vi "ScoreControl.vi"(0 "Get/Set Mode Selector":u16(ring) items=["Get All", "Set", "Reset All", "Force Set", "Force Set All"], 5 "Full Score Entry":T3={"Elements"=[{"Name"="CO2 Balls Touching/Within Reservoir Model", "Value"="-1"}, {"Name"="Money Ball Touching/Within Reservoir Model", "Value"="-1"}, {"Name"="3+ Red/White Citizens in Pink Grid Area", "Value"="-1"}, {"Name"="# Upright Levee Blocks touching ONLY GREEN shores", "Value"="-1"}, {"Name"="# Upright Levee Blocks Touching any RED shore", "Value"="-1"}, {"Name"="Levee Test was Performed", "Value"="-1"}, {"Name"="Levee Test Wheel Blocked by NonLevee", "Value"="-1"}, {"Name"="Flood Barrier in Up Position", "Value"="-1"}, {"Name"="Both Yellow Arrows Aligned", "Value"="-1"}, {"Name"="Team Robot Touching Only Yellow Grid Area", "Value"="-1"}, {"Name"="Both Insulation Touching Green Grid Area", "Value"="-1"}, {"Name"="Bicycle Touching Green Grid Area", "Value"="-1"}, {"Name"="Computer Touching Green Grid Area", "Value"="-1"}, {"Name"="House in Up Position", "Value"="-1"}, {"Name"="House Window Showing Black", "Value"="-1"}, {"Name"="House Window All The Way Open", "Value"="-1"}, {"Name"="3+ Black/White Scientists Touching Research Area", "Value"="-1"}, {"Name"="Money Ball Touching/Within Research Area Model", "Value"="-1"}, {"Name"="Polar Bear Touching/Within Research Area Model", "Value"="-1"}, {"Name"="Polar Bear Orientation (Sleeping/Upright)", "Value"="-1"}, {"Name"="Ice Core Pulled From Its Hole", "Value"="-1"}, {"Name"="Ice Buoy Upright and Within/Touching Research Area Model", "Value"="-1"}, {"Name"="Drilling Machine Touching/Within Research Area Model", "Value"="-1"}, {"Name"="Drill Assembly Completely Vertical", "Value"="-1"}, {"Name"="Team Robot Touching/Within Research Area Model", "Value"="-1"}, {"Name"="3+ Blue/Gray Leaders Touching Green Mountain/City Area", "Value"="-1"}, {"Name"="Ice Core in Base Area", "Value"="-1"}, {"Name"="Snowmobile Touching/Within Research Area Model", "Value"="-1"}], "Score"=0.0}, 7 "GUID":u16, 9 "Round Number":u16, 11 "Score Mode Selector":u16(ring) items=["Automatic", "Manual"], 12 "All Scores":T1 {"Score"."Score Mode Selector" items=["Automatic", "Manual"]}) -> (4 "Scores":T1 {"Score"."Score Mode Selector" items=["Automatic", "Manual"]}, 15 "Errors":string)   [LabVIEW 2013]
uses:
  ScoreEntry.ctl
  ScoreList.ctl
  Full Score Entry.ctl
  Score Event Refnum.vi
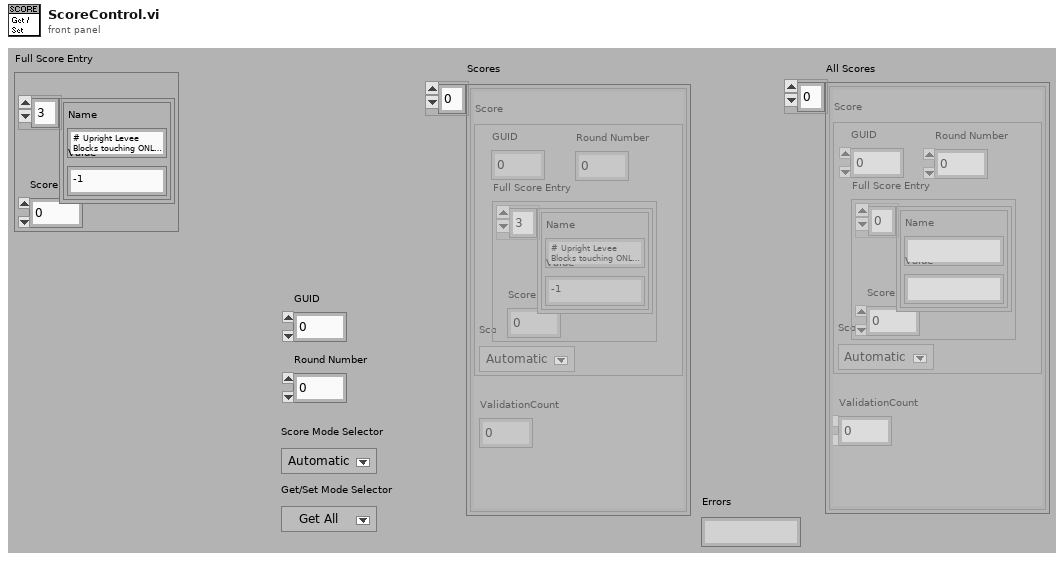
[diagram p1: front panel]
types:
  T1 = typedef "ScoreList.ctl" = cluster{"ValidationCount":u16, "Score":T2}[]
  T2 = typedef "Full Score Entry.ctl" = cluster{"GUID":u16, "Score Mode Selector":u16, "Round Number":u16, "Full Score Entry":T3}
  T3 = typedef "ScoreEntry.ctl" = cluster{"Elements":cluster{"Name":string, "Value":string}[], "Score":dbl}
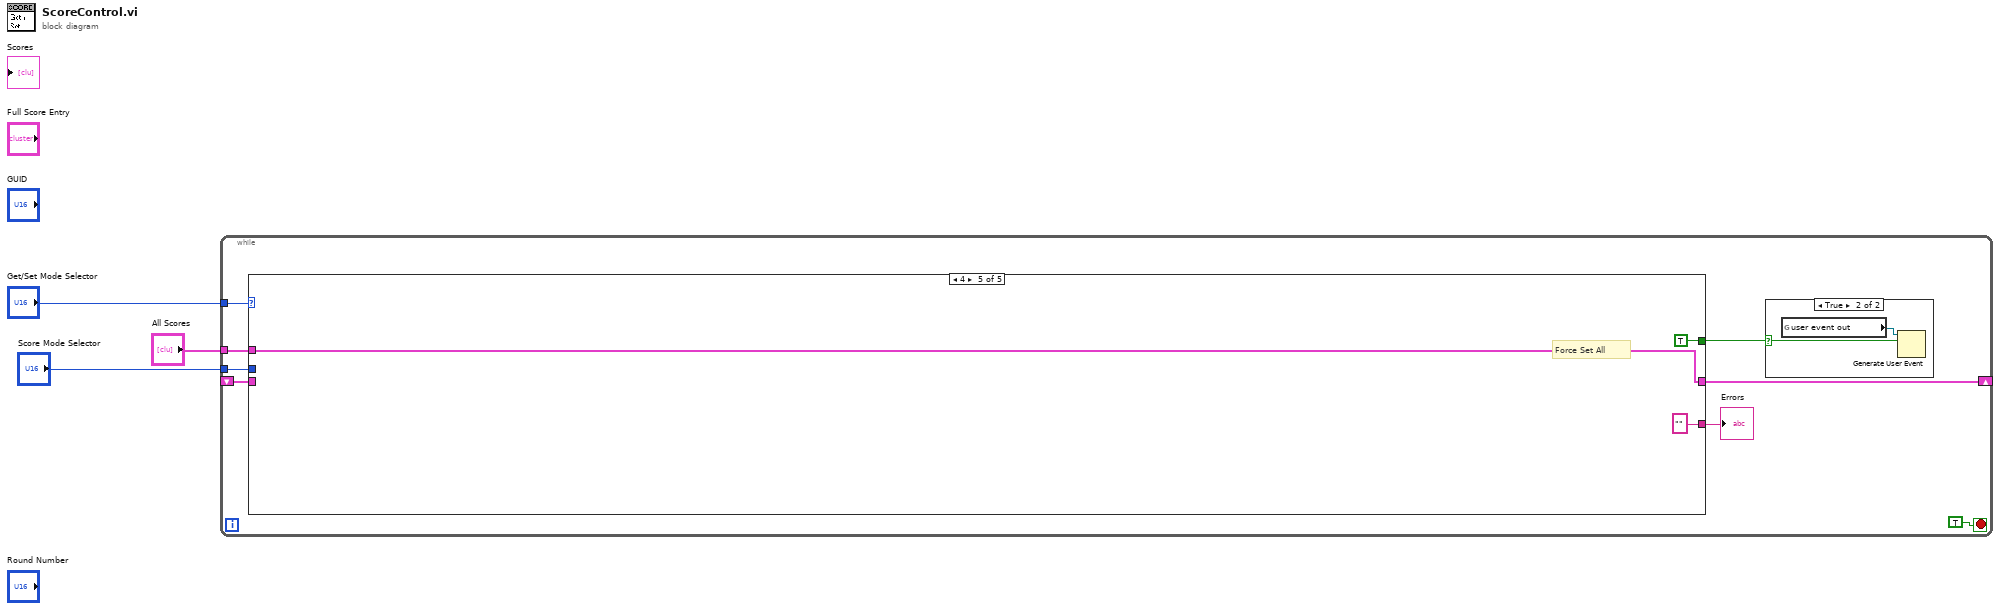
[diagram p0: block diagram]
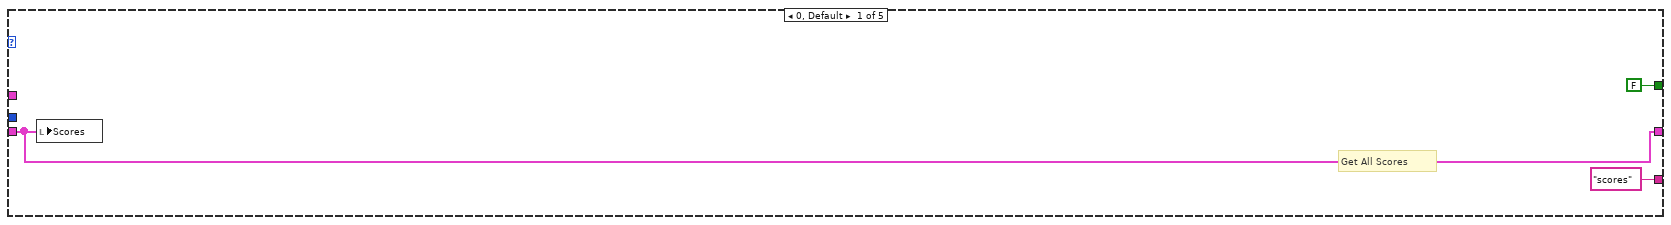
[diagram p3: hidden frame]
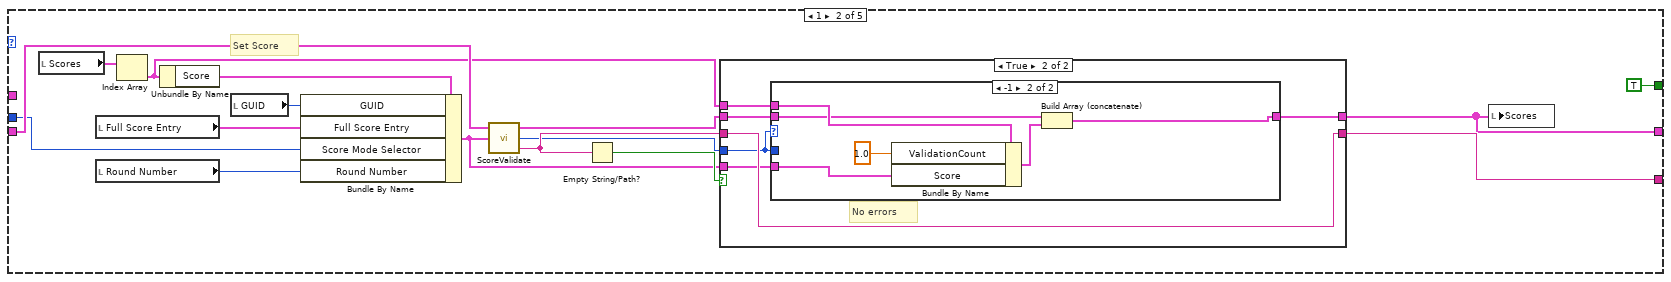
[diagram p4: hidden frame]
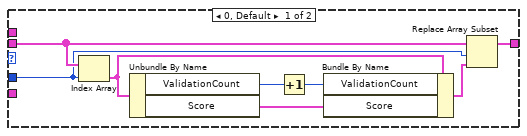
[diagram p6: hidden frame]
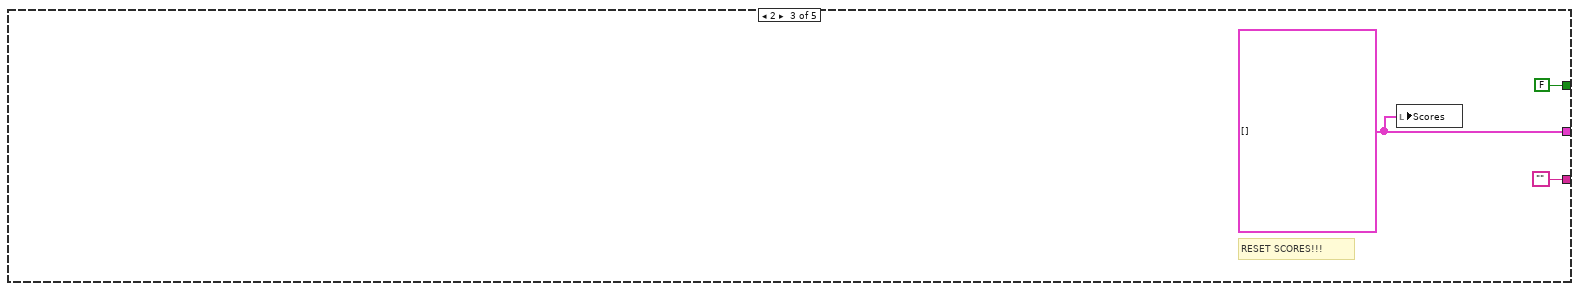
[diagram p7: hidden frame]
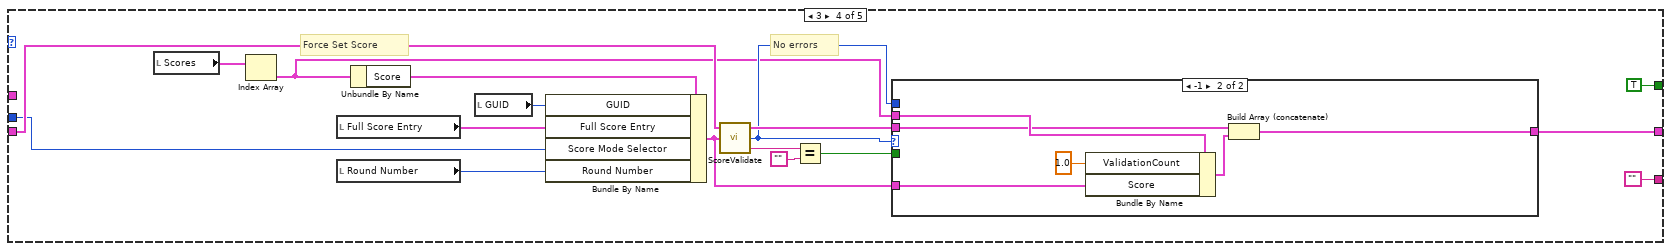
[diagram p8: hidden frame]
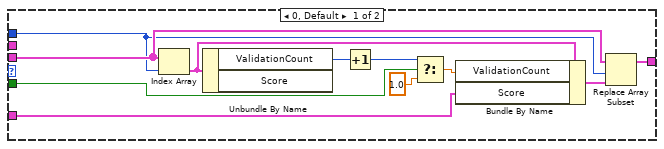
[diagram p9: hidden frame]
diagram:
  n1 = while {
    tunnel: "Get/Set Mode Selector" -> [w11]
    tunnel: "Score Mode Selector" -> [w10]
    shift-right: [w7] -> _
    shift-left: _ -> [w9]
    tunnel: "All Scores" -> [w6]
    stop <- TRUE stop-if-true
    n2 = case shown="4" w11 {
      tunnel: w9 -> [w16 w32 _ w74 _]
      tunnel: [w16 w18 w56 w66 w92] -> w7
      tunnel: ["scores" w31 "" "" "" ("Errors")] -> w5
      tunnel: w10 -> [_ w19 _ w62 _]
      tunnel: w6 -> [_ _ _ _ w92]
      tunnel: [FALSE ("event data") TRUE ("event data") FALSE ("event data") TRUE ("event data") TRUE ("event data")] -> w4
      frame 0, Default {
        # "Get All Scores"
        n3 = local write "Scores"(w16) -> ()
      }
      frame 1 {
        # "Set Score"
        n4 = local read "Scores"() -> (w30:T1)
        n5 = local read "Full Score Entry"() -> (w29:T3)
        n6 = local read "Round Number"() -> (w27:u16)
        n7 = Index Array(array=w30) -> (element=w20:cluster{"ValidationCount":u16, "Score":T2})  [unwired: 1 in]
        n8 = Unbundle By Name(w20) -> ("Score"=w22:T2)
        n9 = local read "GUID"() -> (w28:u16)
        n10 = Bundle By Name(cluster=w22, "GUID"=w28, "Full Score Entry"=w29, "Score Mode Selector"=w19, "Round Number"=w27) -> (w24:T2)
        n11 = call "ScoreValidate.vi"("Score"=w24, "Scores"=w32) -> ("Errors"=w23:string, "Index"=w21:i32, "Scores Out"=w25:T1)  [unwired: 1 in]
        n12 = Empty String/Path?(string/path=w23) -> (empty?=w26:bool)
        n13 = case shown="True" w26 {
          tunnel: w25 -> [w33 w38]
          tunnel: w24 -> [_ w36]
          tunnel: w23 -> [w34 w40]
          tunnel: [w34 w40] -> w31
          tunnel: [w33 w39] -> w18
          tunnel: w21 -> [_ w37]
          tunnel: w20 -> [_ w35]
          frame False {
          }
          frame True {
            # "No errors"
            n14 = case shown="-1" w37 {
              tunnel: [w48 w49] -> w39
              tunnel: w38 -> [w47 w50]
              tunnel: w37 -> [w41 _]
              tunnel: w36 -> [_ w53]
              tunnel: w35 -> [_ w52]
              frame 0, Default {
                n15 = Index Array(array=w47, index=w41) -> (element=w46:cluster{"ValidationCount":u16, "Score":T2})
                n16 = Unbundle By Name(w46) -> ("ValidationCount"=w43:u16, "Score"=w42:T2)
                n17 = Increment(x=w43) -> (x+1=w44:u16)
                n18 = Bundle By Name(cluster=w46, "ValidationCount"=w44, "Score"=w42) -> (w45:cluster{"ValidationCount":u16, "Score":T2})
                n19 = Replace Array Subset(array=w47, new element=w45, index=w41) -> (w48:T1)
              }
              frame -1 {
                n20 = Bundle By Name(cluster=w52, "ValidationCount"=1.0, "Score"=w53) -> (w51:cluster{"ValidationCount":u16, "Score":T2})
                n21 = Build Array (concatenate)(w50, w51) -> (w49:T1)
              }
            }
          }
        }
        n22 = local write "Scores"(w18) -> ()
      }
      frame 2 {
        w56 = T1 [] ("Scores")
        # "RESET SCORES!!!"
        n23 = local write "Scores"(w56) -> ()
      }
      frame 3 {
        # "No errors"
        # "Force Set Score"
        n24 = local read "Scores"() -> (w73:T1)
        n25 = Index Array(array=w73) -> (element=w64:cluster{"ValidationCount":u16, "Score":T2})  [unwired: 1 in]
        n26 = local read "Full Score Entry"() -> (w72:T3)
        n27 = local read "Round Number"() -> (w70:u16)
        n28 = Unbundle By Name(w64) -> ("Score"=w67:T2)
        n29 = local read "GUID"() -> (w71:u16)
        n30 = Bundle By Name(cluster=w67, "GUID"=w71, "Full Score Entry"=w72, "Score Mode Selector"=w62, "Round Number"=w70) -> (w68:T2)
        n31 = call "ScoreValidate.vi"("Score"=w68, "Scores"=w74) -> ("Errors"=w61:string, "Index"=w65:i32, "Scores Out"=w69:T1)  [unwired: 1 out]
        n32 = Equal?(x=w61, y="") -> (x = y?=w59:bool)
        n33 = case shown="-1" w65 {
          tunnel: [w85 w86] -> w66
          tunnel: w69 -> [w84 w87]
          tunnel: w65 -> [w80 _]
          tunnel: w68 -> [w79 w90]
          tunnel: w64 -> [_ w89]
          tunnel: w59 -> [w77 _]
          frame 0, Default {
            n34 = Index Array(array=w84, index=w80) -> (element=w83:cluster{"ValidationCount":u16, "Score":T2})
            n35 = Unbundle By Name(w83) -> ("ValidationCount"=w81:u16)  [unwired: 1 out]
            n36 = Increment(x=w81) -> (x+1=w76:u16)
            n37 = Select(t=w76, s=w77, f=1.0) -> (s? t:f=w78:dbl)
            n38 = Bundle By Name(cluster=w83, "ValidationCount"=w78, "Score"=w79) -> (w82:cluster{"ValidationCount":u16, "Score":T2})
            n39 = Replace Array Subset(array=w84, new element=w82, index=w80) -> (w85:T1)
          }
          frame -1 {
            n40 = Bundle By Name(cluster=w89, "ValidationCount"=1.0, "Score"=w90) -> (w88:cluster{"ValidationCount":u16, "Score":T2})
            n41 = Build Array (concatenate)(w87, w88) -> (w86:T1)
          }
        }
      }
      frame 4 {
        # "Force Set All"
      }
    }
    "Errors" <- w5
    n42 = case shown="True" w4 {
      selector: w4 -> [_ w12]
      frame False {
      }
      frame True {
        n43 = global read "Score Event Refnum.vi" "user event out"() -> (w13:refnum<user-event>)
        n44 = Generate User Event(user event=w13, event data cluster=w12) -> ()  [unwired: 2 in, 2 out]
      }
    }
  }
